vi "MQTT_Q_Subscribe.vi"(8 "error in (no error)":errorcluster, 10 "Topic":string, 11 "MQTT_Q In":refnum<class "MQTT_Q.lvclass">) -> (0 "error out":errorcluster, 2 "SUBACK Payload":u8[](array[numeric]), 3 "MQTT_Q Out":refnum<class "MQTT_Q.lvclass">)   [LabVIEW 2015, in "MQTT_Q.lvclass"]
uses:
  MQTT_Q.lvclass
  MQTT_Q_PVT_MessageType.ctl
  MQTT_Q_QoS.ctl
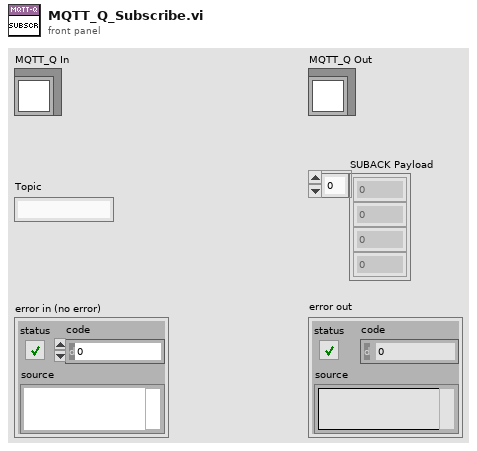
[diagram p1: front panel]
types:
  T1 = typedef "MQTT_Q.lvclass/MQTT_Q_QoS.ctl" = enum8{"At most once", "At least once", "Exactly once", "Reserved"}
  T2 = typedef "MQTT_Q.lvclass/MQTT_Q_PVT_MessageType.ctl" = enum32{"Reserved", "CONNECT", "CONNACK", "PUBLISH", "PUBACK", "PUBREC", "PUBREL", "PUBCOMP", "SUBSCRIBE", "SUBACK", "UNSUBSCRIBE", "UNSUBACK", "PINGREQ", "PINGRESP", "DISCONNECT", "Reserved2"}
  T3 = typedef "MQTT_Q.lvclass/MQTT_Q_PVT_FixedHeader.ctl" = cluster{"MessageType":T2, "DUP Flag":bool, "QoS Level":T1, "RETAIN":bool, "Remaining Length":u32}
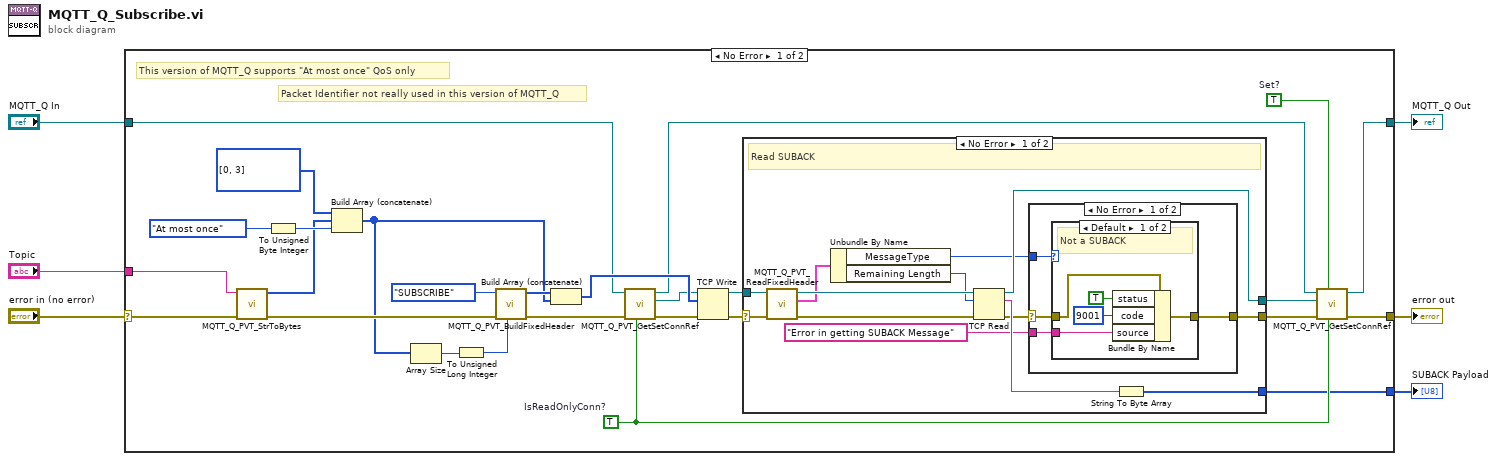
[diagram p0: block diagram]
diagram:
  n1 = case shown="No Error" "error in (no error)" {
    selector: "error in (no error)" -> [w29 w61]
    tunnel: [w24 w61] -> w5
    tunnel: "MQTT_Q In" -> [w22 w60]
    tunnel: [w21 w60] -> w3
    tunnel: "Topic" -> [w9 _]
    tunnel: [w13 _] -> w1
    frame No Error {
      w18 = TRUE  # IsReadOnlyConn?
      w20 = TRUE  # Set?
      # "Packet Identifier not really used in this version of MQTT_Q"
      # "This version of MQTT_Q supports \"At most once\" QoS only"
      n2 = call "MQTT_Q_PVT_StrToBytes.vi"("error in (no error)"=w29, "String in"=w9) -> ("error out"=w28:errorcluster, "Bytes out"=w11:u8[])  [unwired: 8 in]
      n3 = To Unsigned Byte Integer(number=MQTT_Q_QoS."At most once" ("QoS")) -> (unsigned 8bit integer=w12:u8)
      n4 = Build Array (concatenate)(u8[] [0, 3] ("array"), w11, w12) -> (w10:u8[])
      n5 = Array Size(array=w10) -> (size(s)=w31:i32)
      n6 = To Unsigned Long Integer(number=w31) -> (unsigned 32bit integer=w32:u32)
      n7 = call "MQTT_Q_PVT_BuildFixedHeader.vi"("Remaining Length"=w32, "error in (no error)"=w28, "MessageType"=MQTT_Q_PVT_MessageType."SUBSCRIBE") -> ("error out"=w26:errorcluster, "Fixed Header"=w30:u8[])  [unwired: 7 in]
      n8 = Build Array (concatenate)(w30, w10) -> (w27:u8[])
      n9 = call "MQTT_Q_PVT_GetSetConnRef.vi"("IsReadOnlyConn?"=w18, "error in (no error)"=w26, "MQTT_Q in"=w22) -> ("error out"=w25:errorcluster, "connection ID Out"=w19:refnum<k5>, "MQTT_Q out"=w23:refnum<class "MQTT_Q.lvclass">)  [unwired: 6 in]
      n10 = TCP Write(connection ID=w19, data in=w27, error in (no error)=w25) -> (connection ID out=w14:refnum<k5>, error out=w17:errorcluster)  [unwired: 1 in, 1 out]
      n11 = case shown="No Error" w17 {
        selector: w17 -> [w46 w59]
        tunnel: [w36 w59] -> w16
        tunnel: [w43 w58] -> w15
        tunnel: w14 -> [w42 w58]
        tunnel: [w38 _] -> w13
        frame No Error {
          # "Read SUBACK"
          n12 = call "MQTT_Q_PVT_ReadFixedHeader.vi"("error in"=w46, "connection ID"=w42) -> ("error out"=w44:errorcluster, "Fixed Header"=w41:T3, "connection ID out"=w45:refnum<k5>)  [unwired: 6 in, 1 out]
          n13 = Unbundle By Name(w41) -> ("MessageType"=w35:T2, "Remaining Length"=w40:u32)
          n14 = TCP Read(connection ID=w45, bytes to read=w40, error in (no error)=w44) -> (connection ID out=w43:refnum<k5>, data out=w39:string, error out=w37:errorcluster)  [unwired: 2 in]
          n15 = case shown="No Error" w37 {
            selector: w37 -> [w50 w57]
            tunnel: [w48 w57] -> w36
            tunnel: w35 -> [w49 _]
            tunnel: "Error in getting SUBACK Message" ("source") -> [w47 _]
            frame No Error {
              n16 = case shown="Default" w49 {
                tunnel: w50 -> [w55 w56]
                tunnel: [w54 w56] -> w48
                tunnel: w47 -> [w52 _]
                frame Default {
                  # "Not a SUBACK"
                  n17 = Bundle By Name(cluster=w55, "status"=TRUE, "code"=9001, "source"=w52) -> (w54:errorcluster)
                }
                frame "SUBACK" {
                }
              }
            }
            frame Error {
            }
          }
          n18 = String To Byte Array(string=w39) -> (unsigned byte array=w38:u8[])
        }
        frame Error {
        }
      }
      n19 = call "MQTT_Q_PVT_GetSetConnRef.vi"("IsReadOnlyConn?"=w18, "Set?"=w20, "error in (no error)"=w16, "connection ID In"=w15, "MQTT_Q in"=w23) -> ("error out"=w24:errorcluster, "MQTT_Q out"=w21:refnum<class "MQTT_Q.lvclass">)  [unwired: 4 in, 1 out]
    }
    frame Error {
    }
  }
  "error out" <- w5
  "MQTT_Q Out" <- w3
  "SUBACK Payload" <- w1
